vi "LMS Shutdown.vi"(11 "LMS Information Cluster In":T1) -> ()   [LabVIEW 2014]
uses:
  Hokuyo URG Series.lvlib
panel:
  out "Error Out":errorcluster
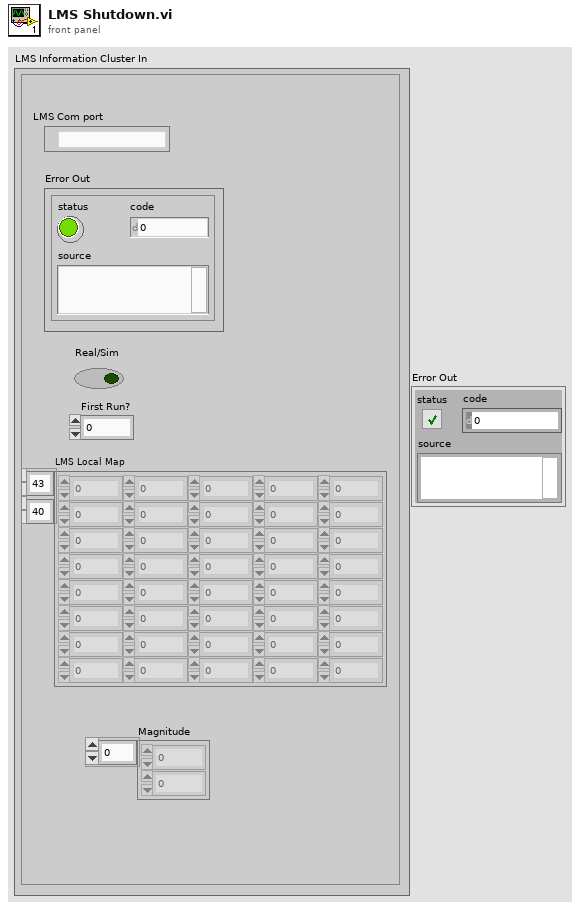
[diagram p1: front panel]
types:
  T1 = cluster{"LMS Com port":refnum<visa-resource-name>, "Error Out":errorcluster, "Real/Sim":bool, "First Run?":i32, "LMS Local Map ":i32[][], "Magnitude":dbl[]}
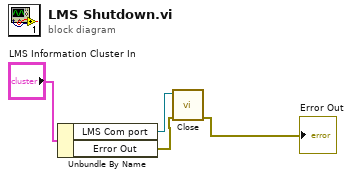
[diagram p0: block diagram]
diagram:
  n1 = Unbundle By Name("LMS Information Cluster In") -> ("LMS Com port"=w3:refnum<visa-resource-name>, "Error Out"=w2:errorcluster)
  n2 = call "Close.vi"("error in (no error)"=w2, "VISA resource name"=w3) -> ("error out"=→"Error Out":errorcluster)  [unwired: 9 in]
